vi "ABB configure Efficiencies.vi"() -> ()   [LabVIEW 2017]
uses:
  ABB global.vi
panel:
  in  "Loads (%Rated)":dbl[](array[numeric]) format="%#.0f"
  in  "Number of Loads":i32
  in  "Exit":bool
  # "Configure Efficiency Report"
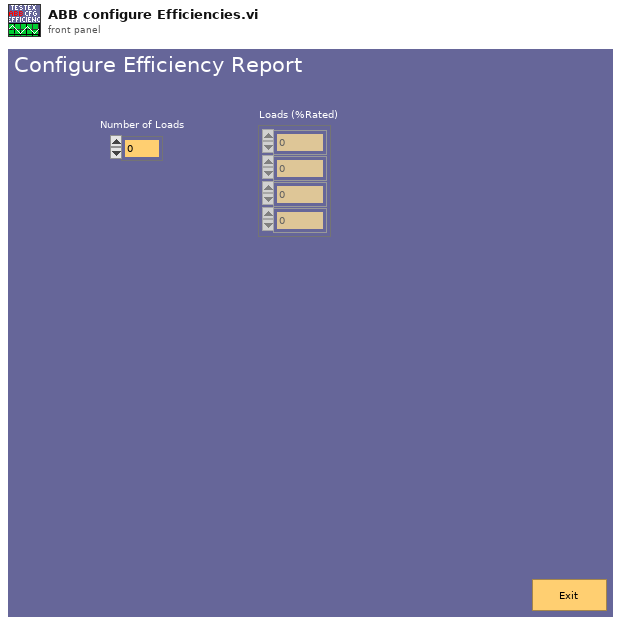
[diagram p1: front panel]
types:
  T1 = cluster{"Number of Loads":i32, "Loads (%Rated)":dbl[]}
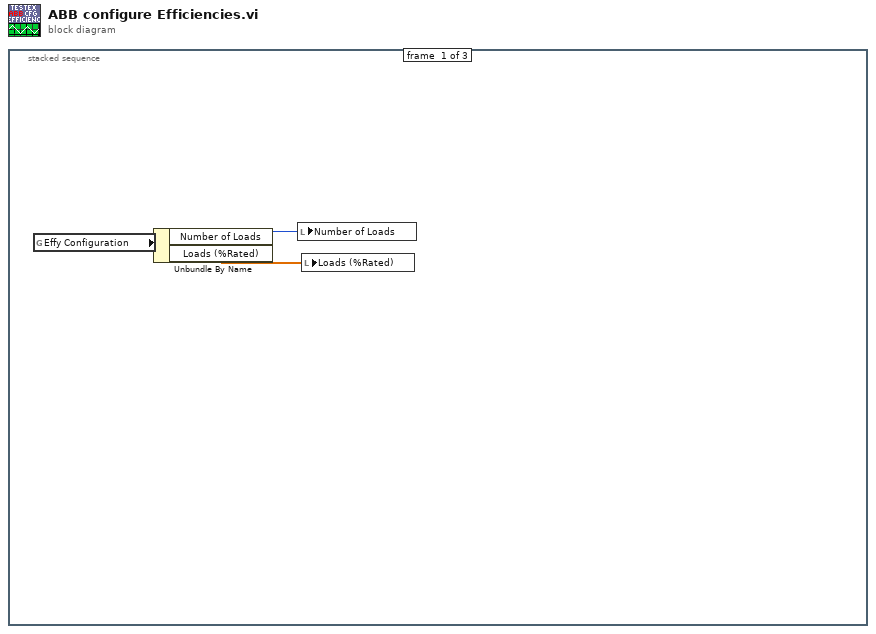
[diagram p0: block diagram]
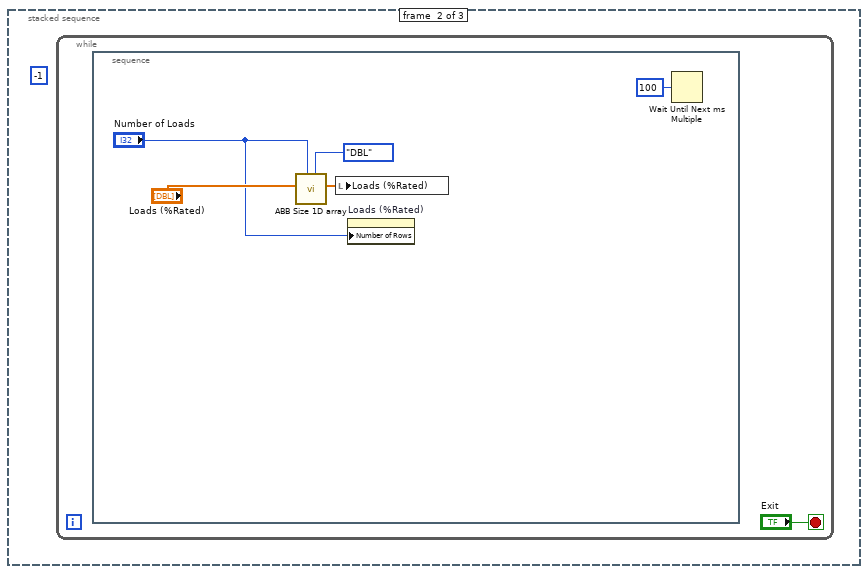
[diagram p2: hidden frame]
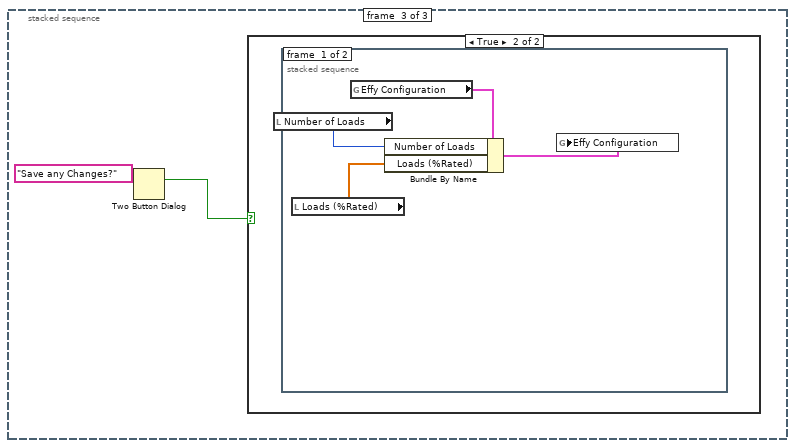
[diagram p3: hidden frame]
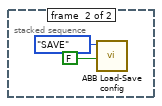
[diagram p5: hidden frame]
diagram:
  n1 = stacked-sequence {
    frame #0 {
      n2 = global read "ABB global.vi" "Effy Configuration"() -> (w3:T1)
      n3 = Unbundle By Name(w3) -> ("Number of Loads"=w2:i32, "Loads (%Rated)"=w1:dbl[])
      n4 = local write "Number of Loads"(w2) -> ()
      n5 = local write "Loads (%Rated)"(w1) -> ()
    }
    frame #1 {
      (unwired) -1 ("Number Values")
      n6 = while {
        stop <- "Exit" stop-if-true
        n7 = stacked-sequence {
          frame #0 {
            n8 = call "ABB Size 1D array.vi"("Type"=enum16{"Integer", "DBL", "STRING", "BOOLEAN"}."DBL", "Size"="Number of Loads", "DBL Array In"="Loads (%Rated)") -> ("DBL Array out"=w7:dbl[])  [unwired: 5 in, 3 out]
            n9 = local write "Loads (%Rated)"(w7) -> ()
            n10 = property on="Loads (%Rated)" class="Arr (strict)"("Number of Rows"="Number of Loads") -> ()  [unwired: 2 in, 2 out]
            n11 = Wait Until Next ms Multiple(millisecond multiple=u32 100) -> ()  [unwired: 1 out]
          }
        }
      }
    }
    frame #2 {
      n12 = Two Button Dialog(message="Save any Changes?") -> (T button?=w11:bool)  [unwired: 2 in]
      n13 = case shown="True" w11 {
        frame False {
        }
        frame True {
          n14 = stacked-sequence {
            frame #0 {
              n15 = local read "Number of Loads"() -> (w13:i32)
              n16 = local read "Loads (%Rated)"() -> (w12:dbl[])
              n17 = global read "ABB global.vi" "Effy Configuration"() -> (w15:T1)
              n18 = Bundle By Name(cluster=w15, "Number of Loads"=w13, "Loads (%Rated)"=w12) -> (w14:T1)
              n19 = global write "ABB global.vi" "Effy Configuration"(w14) -> ()
            }
            frame #1 {
              n20 = call "ABB Load-Save config.vi"("confirm save"=FALSE, "Mode"=enum16{"LOAD", "SAVE"}."SAVE") -> ()  [unwired: 10 in]
            }
          }
        }
      }
    }
  }
